vi "Scripting_AssignControlToConnectorPane.vi"() -> ()   [LabVIEW 2020]
uses:
  Scripting_ConnectorPanePatternType.ctl
  Scripting_FollowWireDownStreams_StopCriteria.ctl
  Scripting.lvclass
  Scripting_NodeInfo.ctl
  Scripting_ObjectType.ctl
  Scripting_PastThroughObjectType.ctl
  SubVIs/Scripting_ViDependencyType.ctl
  Scripting_VIClassDependency.ctl
panel:
  in  "error in (no error)":errorcluster
  in  "VI-Path/VI-Ref":variant
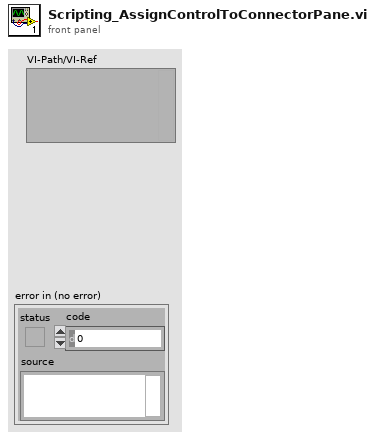
[diagram p1: front panel]
types:
  T1 = typedef "LVRectTypeDef.ctl" = cluster{"Left":i16, "Top":i16, "Right":i16, "Bottom":i16}
  T2 = typedef "Scripting_VIClassDependency.ctl" = cluster{"VIPath":path, "Class":string, "ClassPath":path, "ViDependencyType":T3}
  T3 = typedef "Scripting_ViDependencyType.ctl" = enum16{"N/A", "Launches"}
  T4 = typedef "Scripting.lvclass/Scripting_PastThroughObjectType.ctl" = cluster{"Object":refnum<vi>, "InsideArray":bool, "PastThroughObjectTypes":T5[], "ObjectType":string, "ObjectData":string}
  T5 = typedef "Scripting_ObjectType.ctl" = cluster{"ObjectType":string, "ObjectName":string, "ObjectTerminalName":string}
  T6 = typedef "Scripting_NodeInfo.ctl" = cluster{"Type":string, "Style":string, "ObjectRef":refnum<vi>, "Terms":refnum<vi>[], "Sources":refnum<vi>[], "Drains":refnum<vi>[], "DrainsSourcesTerms":refnum<vi>[], "SourcesDrainTerms":cluster{"DrainsTerms":refnum<vi>[]}[], "UpperLeftPosition":cluster{"Left":i32, "Top":i32}, "LowerRightPosition":cluster{"Right":i32, "Bottom":i32}}
  T7 = typedef "Scripting_FollowWireDownStreams_StopCriteria.ctl" = cluster{"ReachedANyOfTheseNodes":refnum<vi>[], "NodeType":string[], "VINames":string[], "AddTheseNodes":bool, "ALsoSerachOtherDrainNodes":bool}
  T8 = typedef "Scripting_ConnectorPanePatternType.ctl" = u16
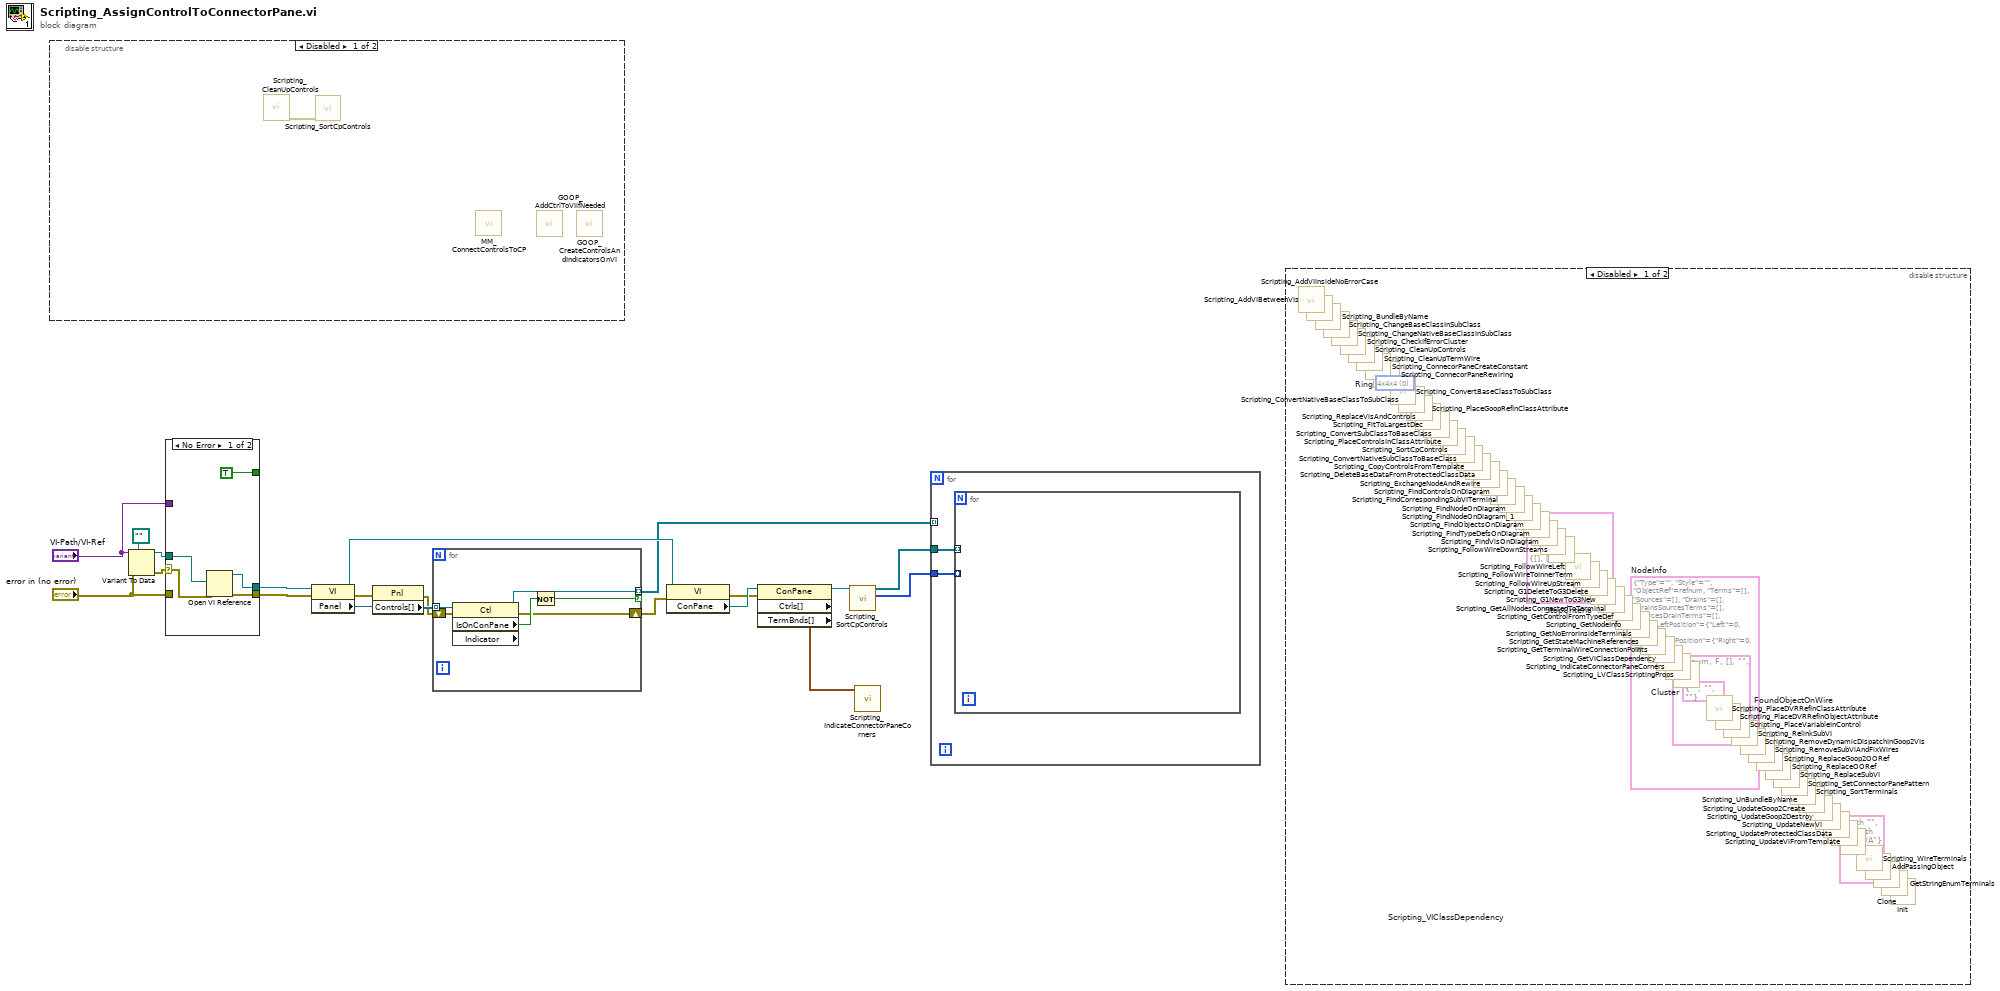
[diagram p0: block diagram]
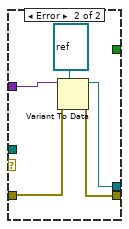
[diagram p3: hidden frame]
diagram:
  n1 = disable-structure shown="Disabled" {
    frame Disabled {
      n2 = call "Scripting_CleanUpControls.vi"() -> ("error out"=w21:errorcluster)  [unwired: 10 in, 1 out]
      n3 = call "Scripting_SortCpControls.vi"("error in (no error)"=w21) -> ()  [unwired: 4 in, 7 out]
      n4 = call "MM_ConnectControlsToCP.vi"() -> ()  [unwired: 10 in, 2 out]
      n5 = call "GOOP_AddCtrlToVIIfNeeded.vi"() -> ()  [unwired: 9 in, 3 out]
      n6 = call "GOOP_CreateControlsAndIndicatorsOnVI.vi"() -> ()  [unwired: 11 in, 1 out]
    }
    frame Enabled {
    }
  }
  n7 = Variant To Data(error in="error in (no error)", type=path "" ("vi path"), Variant="VI-Path/VI-Ref") -> (data=w14:path, error out=w13:errorcluster)
  n8 = case shown="No Error" w13 {
    selector: w13 -> [w23 _]
    tunnel: [w24 w29] -> w20
    tunnel: "error in (no error)" -> [_ w27]
    tunnel: [w26 w28] -> w18
    tunnel: w14 -> [w25 _]
    tunnel: "VI-Path/VI-Ref" -> [_ w31]
    tunnel: [TRUE _] -> _
    frame No Error {
      n9 = Open VI Reference(vi path=w25, error in (no error)=w23) -> (vi reference=w24:refnum<vi>, error out=w26:errorcluster)  [unwired: 4 in]
    }
    frame Error {
      n10 = Variant To Data(error in=w27, type=refnum<vi> refnum ("reference"), Variant=w31) -> (data=w29:refnum<vi>, error out=w28:errorcluster)
    }
  }
  n11 = property class="VI"(reference=w20, error in=w18) -> (reference out=w8:refnum<vi>, error out=w9:errorcluster, "Panel"=w10:refnum<vi>)
  n12 = property class="Pnl"(reference=w10, error in=w9) -> (error out=w6:errorcluster, "Controls[]"=w7:refnum<vi>[])  [unwired: 1 out]
  n13 = for {
    tunnel: w7 -> [w37] mode=indexing
    tunnel: [w36] -> w3 mode=indexing if=w34
    shift-right: [w32] -> w5
    shift-left: w6 -> [w33]
    n14 = property class="Ctl" props=["IsOnConPane", "Indicator"](reference=w37, error in=w33) -> (reference out=w36:refnum<vi>, error out=w32:errorcluster, "IsOnConPane"=w35:bool)  [unwired: 1 out]
    n15 = Not(x=w35) -> (.not. x?=w34:bool)
  }
  n16 = property class="VI"(reference=w8, error in=w5) -> (error out=w17:errorcluster, "ConPane"=w19:refnum<vi>)  [unwired: 1 out]
  n17 = property class="ConPane" props=["Ctrls[]", "TermBnds[]"](reference=w19, error in=w17) -> (reference out=w4:refnum<vi>, "TermBnds[]"=w16:T1[])  [unwired: 2 out]
  n18 = call "Scripting_SortCpControls.vi"("Connector Pane:Reference"=w4) -> ("TermIndex"=w1:i32[], "Controls[]"=w2:refnum<vi>[])  [unwired: 4 in, 5 out]
  n19 = call "Scripting_IndicateConnectorPaneCorners.vi"("TermBnds[]"=w16) -> ()  [unwired: 7 in, 4 out]
  n20 = for {
    tunnel: w3 -> [_] mode=indexing
    tunnel: w2 -> [w39]
    tunnel: w1 -> [w38]
    n21 = for {
      tunnel: w39 -> [_] mode=indexing
      tunnel: w38 -> [_] mode=indexing
    }
  }
  n22 = disable-structure shown="Disabled" {
    frame Disabled {
      (unwired) T2 {"VIPath"=path "", "Class"="", "ClassPath"=path "", "ViDependencyType"=enum."N/A"}  # Scripting_VIClassDependency
      (unwired) T4 {"Object"=refnum, "InsideArray"=FALSE, "PastThroughObjectTypes"=[], "ObjectType"="", "ObjectData"=""}  # FoundObjectOnWire
      (unwired) T5 {"ObjectType"="", "ObjectName"="", "ObjectTerminalName"=""}  # Cluster
      (unwired) T6 {"Type"="", "Style"="", "ObjectRef"=refnum, "Terms"=[], "Sources"=[], "Drains"=[], "DrainsSourcesTerms"=[], "SourcesDrainTerms"=[], "UpperLeftPosition"={"Left"=0, "Top"=0}, "LowerRightPosition"={"Right"=0, "Bottom"=0}}  # NodeInfo
      (unwired) T7 {"ReachedANyOfTheseNodes"=[], "NodeType"=[], "VINames"=[], "AddTheseNodes"=FALSE, "ALsoSerachOtherDrainNodes"=FALSE}  # StopCriteria
      (unwired) T8 0 items=["4x4x4", "5x6x5", "6x8x6"]  # Ring
      n23 = call "Scripting_AddVIBetweenVIs.vi"() -> ()  [unwired: 18 in, 2 out]
      n24 = call "Scripting_AddVIInsideNoErrorCase.vi"() -> ()  [unwired: 19 in, 1 out]
      n25 = call "Scripting_BundleByName.vi"() -> ()  [unwired: 19 in, 1 out]
      n26 = call "Scripting_ChangeBaseClassInSubClass.vi"() -> ()  [unwired: 19 in, 1 out]
      n27 = call "Scripting_ChangeNativeBaseClassInSubClass.vi"() -> ()  [unwired: 19 in, 1 out]
      n28 = call "Scripting_CheckIfErrorCluster.vi"() -> ()  [unwired: 9 in, 3 out]
      n29 = call "Scripting_CleanUpControls.vi"() -> ()  [unwired: 10 in, 2 out]
      n30 = call "Scripting_CleanUpTermWire.vi"() -> ()  [unwired: 10 in, 2 out]
      n31 = call "Scripting_ConnecorPaneCreateConstant.vi"() -> ()  [unwired: 19 in, 1 out]
      n32 = call "Scripting_ConnecorPaneRewiring.vi"() -> ()  [unwired: 19 in, 1 out]
      n33 = call "Scripting_ConvertBaseClassToSubClass.vi"() -> ()  [unwired: 19 in, 1 out]
      n34 = call "Scripting_ConvertNativeBaseClassToSubClass.vi"() -> ()  [unwired: 19 in, 1 out]
      n35 = call "Scripting_PlaceGoopRefInClassAttribute.vi"() -> ()  [unwired: 4 in, 4 out]
      n36 = call "Scripting_ReplaceVisAndControls.vi"() -> ()  [unwired: 18 in, 2 out]
      n37 = call "Scripting_FitToLargestDec.vi"() -> ()  [unwired: 6 in, 2 out]
      n38 = call "Scripting_ConvertSubClassToBaseClass.vi"() -> ()  [unwired: 19 in, 1 out]
      n39 = call "Scripting_PlaceControlsInClassAttribute.vi"() -> ()  [unwired: 13 in, 3 out]
      n40 = call "Scripting_SortCpControls.vi"() -> ()  [unwired: 5 in, 7 out]
      n41 = call "Scripting_ConvertNativeSubClassToBaseClass.vi"() -> ()  [unwired: 19 in, 1 out]
      n42 = call "Scripting_CopyControlsFromTemplate.vi"() -> ()  [unwired: 19 in, 1 out]
      n43 = call "Scripting_DeleteBaseDataFromProtectedClassData.vi"() -> ()  [unwired: 19 in, 1 out]
      n44 = call "Scripting_ExchangeNodeAndRewire.vi"() -> ()  [unwired: 19 in, 1 out]
      n45 = call "Scripting_FindControlsOnDiagram.vi"() -> ()  [unwired: 17 in, 3 out]
      n46 = call "Scripting_FindCorrespondingSubVITerminal.vi"() -> ()  [unwired: 13 in, 7 out]
      n47 = call "Scripting_FindNodeOnDiagram.vi"() -> ()  [unwired: 18 in, 2 out]
      n48 = call "Scripting_FindNodeOnDiagram_1.vi"() -> ()  [unwired: 18 in, 2 out]
      n49 = call "Scripting_FindObjectsOnDiagram.vi"() -> ()  [unwired: 18 in, 2 out]
      n50 = call "Scripting_FindTypeDefsOnDiagram.vi"() -> ()  [unwired: 18 in, 2 out]
      n51 = call "Scripting_FindVisOnDiagram.vi"() -> ()  [unwired: 18 in, 2 out]
      n52 = call "Scripting_FollowWireDownStreams.vi"() -> ()  [unwired: 16 in, 4 out]
      n53 = call "Scripting_FollowWireLeft.vi"() -> ()  [unwired: 16 in, 4 out]
      n54 = call "Scripting_FollowWireToInnerTerm.vi"() -> ()  [unwired: 18 in, 2 out]
      n55 = call-dynamic "Scripting_FollowWireUpStream.vi"() -> ()  [unwired: 18 in, 2 out]
      n56 = call "Scripting_G1DeleteToG3Delete.vi"() -> ()  [unwired: 19 in, 1 out]
      n57 = call "Scripting_G1NewToG3New.vi"() -> ()  [unwired: 19 in, 1 out]
      n58 = call "Scripting_GetAllNodesConnectedToTerminal.vi"() -> ()  [unwired: 16 in, 4 out]
      n59 = call "Scripting_GetControlFromTypeDef.vi"() -> ()  [unwired: 16 in, 4 out]
      n60 = call "Scripting_GetNodeInfo.vi"() -> ()  [unwired: 17 in, 3 out]
      n61 = call "Scripting_GetNoErrorInsideTerminals.vi"() -> ()  [unwired: 13 in, 7 out]
      n62 = call "Scripting_GetStateMachineReferences.vi"() -> ()  [unwired: 1 in]
      n63 = call "Scripting_GetTerminalWireConnectionPoints.vi"() -> ()  [unwired: 11 in, 9 out]
      n64 = call "Scripting_GetVIClassDependency.vi"() -> ()  [unwired: 18 in, 2 out]
      n65 = call "Scripting_IndicateConnectorPaneCorners.vi"() -> ()  [unwired: 8 in, 4 out]
      n66 = call "Scripting_LVClassScriptingProps.vi"() -> ()  [unwired: 1 in]
      n67 = call "Scripting_PlaceDVRRefInClassAttribute.vi"() -> ()  [unwired: 4 in, 4 out]
      n68 = call "Scripting_PlaceDVRRefInObjectAttribute.vi"() -> ()  [unwired: 19 in, 1 out]
      n69 = call "Scripting_PlaceVariableInControl.vi"() -> ()  [unwired: 15 in, 1 out]
      n70 = call "Scripting_RelinkSubVI.vi"() -> ()  [unwired: 10 in, 2 out]
      n71 = call "Scripting_RemoveDynamicDispatchInGoop2VIs.vi"() -> ()  [unwired: 18 in, 2 out]
      n72 = call "Scripting_RemoveSubViAndFixWires.vi"() -> ()  [unwired: 19 in, 1 out]
      n73 = call "Scripting_ReplaceGoop2OORef.vi"() -> ()  [unwired: 19 in, 1 out]
      n74 = call "Scripting_ReplaceOORef.vi"() -> ()  [unwired: 19 in, 1 out]
      n75 = call "Scripting_ReplaceSubVI.vi"() -> ()  [unwired: 10 in, 2 out]
      n76 = call "Scripting_SetConnectorPanePattern.vi"() -> ()  [unwired: 19 in, 1 out]
      n77 = call "Scripting_SortTerminals.vi"() -> ()  [unwired: 9 in, 3 out]
      n78 = call "Scripting_UnBundleByName.vi"() -> ()  [unwired: 19 in, 1 out]
      n79 = call "Scripting_UpdateGoop2Create.vi"() -> ()  [unwired: 19 in, 1 out]
      n80 = call "Scripting_UpdateGoop2Destroy.vi"() -> ()  [unwired: 19 in, 1 out]
      n81 = call "Scripting_UpdateNewVI.vi"() -> ()  [unwired: 19 in, 1 out]
      n82 = call "Scripting_UpdateProtectedClassData.vi"() -> ()  [unwired: 10 in, 2 out]
      n83 = call "Scripting_UpdateViFromTemplate.vi"() -> ()  [unwired: 18 in, 2 out]
      n84 = call "Scripting_WireTerminals.vi"() -> ()  [unwired: 11 in, 1 out]
      n85 = call "AddPassingObject.vi"() -> ()  [unwired: 18 in, 2 out]
      n86 = call-dynamic "Clone.vi"() -> ()  [unwired: 18 in, 2 out]
      n87 = call "GetStringEnumTerminals.vi"() -> ()  [unwired: 10 in, 2 out]
      n88 = call "Init.vi"() -> ()  [unwired: 18 in, 2 out]
    }
    frame Enabled {
    }
  }
